vi "Drive Until Distance with Vision.vi"(11 "Distance Set Point":dbl) -> (3 "Done?":bool)   [LabVIEW 2016]
uses:
  Robot Values.vi
  <vilib>/addons/control/pid/pid.llb/PID (DBL).vi
  Vision Global.vi
  <vilib>/addons/control/pid/NI_PID_pid.lvlib
  <vilib>/ptbypt/NI_PtbyPt.lvlib
panel:
  in  "Time Tolerance":dbl=0.15 format="%#_13g"
  out "Elapsed Time (s)":dbl
  in  "Error PID gains":T1={"proportional gain (Kc)"=0.65, "integral time (Ti, min)"=0.0, "derivative time (Td, min)"=0.0} {"derivative time (Td, min)" format="%.3f"; "integral time (Ti, min)" format="%.3f"; "proportional gain (Kc)" format="%.3f"}
  in  "PID gains":T1={"proportional gain (Kc)"=1.0, "integral time (Ti, min)"=0.0, "derivative time (Td, min)"=0.0} {"derivative time (Td, min)" format="%.3f"; "integral time (Ti, min)" format="%.3f"; "proportional gain (Kc)" format="%.3f"}
  # "Comp:\n.042\n0\n0"
  # "Comp:\n.1\n0\n0"
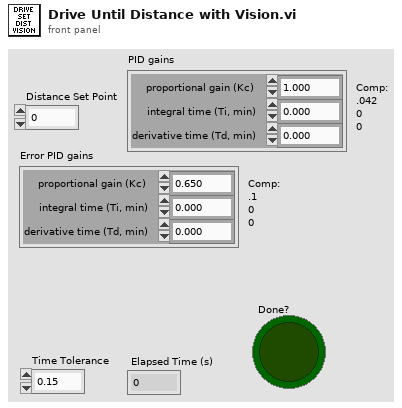
[diagram p1: front panel]
types:
  T1 = cluster{"proportional gain (Kc)":dbl, "integral time (Ti, min)":dbl, "derivative time (Td, min)":dbl}
  T2 = typedef "Robot Values.ctl" = cluster{"Robot Drive":cluster{"Left Motor Power":dbl, "Right Motor Power":dbl, "Left Encoder Value":dbl, "Right Encoder Value":dbl, "High Gear?":bool, "PTO?":bool}, "Sensors":cluster{"Gyro Angle":u16, "Recalibrate Gyro":bool, "Reset Gyro":bool, "Ultrasonic":dbl}, "Shooter":cluster{"Prep Wheels":bool, "Shoot":bool, "Left Shooter Wheel Speed":dbl, "Wheels Moving":bool, "Shooter Prepped":bool, "Shooter RPS SP":dbl, "Shooting?":bool, "Left Shooter Wheel Power":dbl, "Right Shooter Wheel Power":dbl, "Acquisition Conveyor Power":dbl, "Hopper Beater Bar Power":dbl, "Filtered Left Shooter Speed":dbl, "Acquisition Motor Power":dbl, "Joystick Add":dbl}, "Robot States":cluster{"Drive mode":string, "Alliance":T3, "Position":T4}, "Gear":cluster{"Ejection Active":bool}}
  T3 = typedef "WPI_DriverStationAllianceInfo.ctl" = enum16{"Red", "Blue", "Invalid"}
  T4 = typedef "WPI_DriverStationPositionInfo.ctl" = enum16{"1", "2", "3"}
  T5 = cluster{"Distance (ft)":dbl, "Score":dbl, "Normalized":cluster{"Center":cluster{dbl, dbl}, "Rectangle":cluster{"Numeric":dbl, "Numeric 2":dbl, "Numeric 3":dbl, "Numeric 5":dbl}}, "Pixels":cluster{"Center":cluster{dbl, dbl}, "Rectangle":cluster{"Numeric":dbl, "Numeric 2":dbl, "Numeric 3":dbl, "Numeric 5":dbl}}}
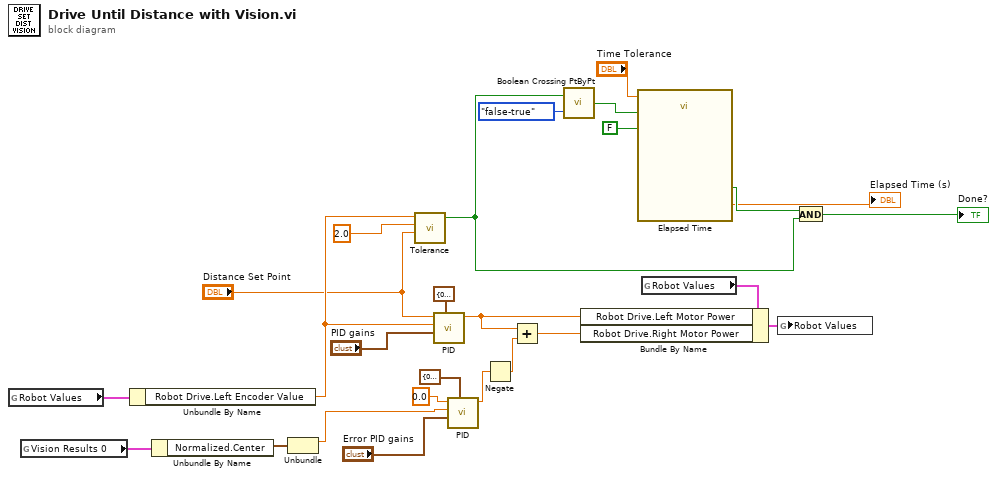
[diagram p0: block diagram]
diagram:
  n1 = global read "Robot Values.vi" "Robot Values"() -> (w26:T2)
  n2 = global read "Vision Global.vi" "Vision Results 0"() -> (w3:T5)
  n3 = Unbundle By Name(w26) -> ("Robot Drive.Left Encoder Value"=w14:dbl)
  n4 = Unbundle By Name(w3) -> ("Normalized.Center"=w2:cluster{dbl, dbl})
  n5 = Unbundle(w2) -> (w1:dbl)  [unwired: 1 out]
  n6 = call "Tolerance.vi"("Setpoint"="Distance Set Point", "Tolerance"=2.0, "Current Value"=w14) -> ("In Range?"=w4:bool)  [unwired: 8 in]
  n7 = call-poly <vilib>:"PID.vi"("output range"=cluster{"output high":dbl, "output low":dbl} {"output high"=0.5, "output low"=-0.5}, "PID gains"="PID gains", "process variable"=w14, "setpoint"="Distance Set Point") -> ("output"=w18:dbl)  [unwired: 6 in, 1 out]
  n8 = call-poly <vilib>:"PID.vi"("output range"=cluster{"output high":dbl, "output low":dbl} {"output high"=0.1, "output low"=-0.1}, "PID gains"="Error PID gains", "process variable"=w1, "setpoint"=0.0) -> ("output"=w16:dbl)  [unwired: 6 in, 1 out]
  n9 = Negate(x=w16) -> (-x=w15:dbl)
  n10 = Add(x=w18, y=w15) -> (x+y=w17:dbl)
  n11 = call <vilib>:"Boolean Crossing PtByPt.vi"("direction"=enum16{"either", "false-true", "true-false"}."false-true", "input"=w4) -> ("crossing"=w9:bool)  [unwired: 1 in]
  n12 = call "Elapsed Time"("Time Target (s)"="Time Tolerance", "Reset"=w9, "Auto Reset"=FALSE) -> ("Elapsed Time (s)"=→"Elapsed Time (s)":dbl, "Time has Elapsed"=w6:bool)  [unwired: 9 in, 6 out]
  n13 = global read "Robot Values.vi" "Robot Values"() -> (w22:T2)
  n14 = Bundle By Name(cluster=w22, "Robot Drive.Left Motor Power"=w18, "Robot Drive.Right Motor Power"=w17) -> (w23:T2)
  n15 = global write "Robot Values.vi" "Robot Values"(w23) -> ()
  n16 = And(x=w6, y=w4) -> (x .and. y?=→"Done?":bool)
